vi "송신2.vi"() -> ()   [LabVIEW 2023]
uses:
  <vilib>/Analysis/NI_AALBase.lvlib
panel:
  in  "Stop Button":bool=TRUE
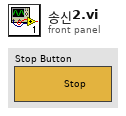
[diagram p1: front panel]
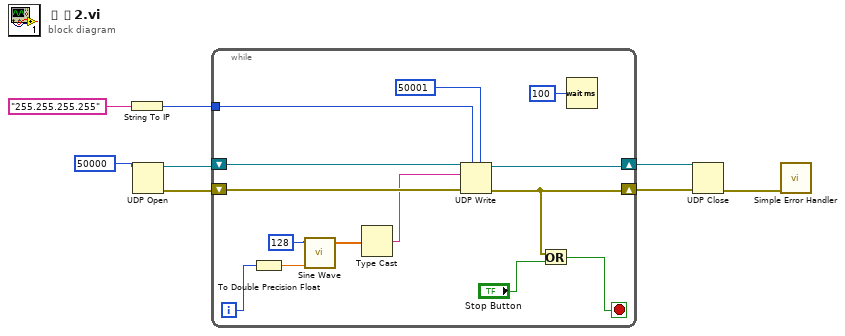
[diagram p0: block diagram]
diagram:
  n1 = String To IP(1:"255.255.255.255" ("Target IP")) -> (0:w4:u32)
  n2 = UDP Open(11:u16 50000 ("port")) -> (port=w6:refnum<k16>, 0:w8:errorcluster)  [unwired: 4 in, 1 out]
  n3 = while {
    shift-right: [w20] -> w5
    shift-left: w6 -> [w21]
    shift-right: [w15] -> w7
    shift-left: w8 -> [w22]
    tunnel: w4 -> [w18]
    i -> [w13]
    stop <- w16 stop-if-true
    n4 = To Double Precision Float(number=w13) -> (double precision float=w12:dbl)
    n5 = call <vilib>:"Sine Wave.vi"("samples"=128, "phase in"=w12) -> ("sine wave"=w11:dbl[])  [unwired: 3 in, 2 out]
    n6 = Type Cast(x=w11) -> (*(type *) &x=w10:string)  [unwired: 1 in]
    n7 = UDP Write(address=w18, port or service name=u16 50001, connection ID=w21, data in=w10, 8:w22) -> (error out=w15:errorcluster, 3:w20:refnum<k16>)  [unwired: 1 in]
    n8 = Or(x=w15, y="Stop Button") -> (x .or. y?=w16:bool)
    n9 = Wait (ms)(milliseconds to wait=u32 100) -> ()  [unwired: 1 out]
  }
  n10 = UDP Close(connection ID=w5, 8:w7) -> (error out=w1:errorcluster)  [unwired: 1 out]
  n11 = call <vilib>:"Simple Error Handler.vi"("error in (no error)"=w1) -> ()  [unwired: 4 in, 5 out]
